vi "FIR calculator.vi"() -> ()   [LabVIEW 2015]
uses:
  <vilib>/measure/NI_MAPro.lvlib
panel:
  out "sum":dbl format="%#_18g"
  in  "COEFFICIENTVECTOR 3":string="-1, 4, 16, 32, -64, 136, -352, 1312,-352, 136, -64, 32, -16, 4, -1"
  out "CIC normalized gain":dbl[](graph)
  in  "Number of stages":i32=3
  in  "CIC input bits":i32
  out "CIC output bits":dbl[](graph)
  out "Waveform Graph 3":cluster{dbl, "df":dbl, "Mag H(w)":dbl[]}(graph)
  in  "COEFFICIENTVECTOR 2":string="-1, 4, 16, 32, -64, 136, -352, 1312,-352, 136, -64, 32, -16, 4, -1"
  out "df":dbl format="%#_6p"
  out "Waveform Graph 2":cluster{dbl, "df":dbl, "Phase H(w)":dbl[]}(graph)
  out "Waveform Graph":cluster{dbl, "df":dbl, "Mag H(w)":dbl[]}(graph)
  out "h":dbl[](array[numeric])
  in  "COEFFICIENTVECTOR1":string="-1.63744122654648e-08, -4.62216716148361e-08, -3.14335779482632e-10, 3.02310153778336e-08, 1.74890850381969e-08, 3.19482286529326e-08, -5.0994421994774e-09, -1.48653353613353e-07, -8.26761935440861e-08, 3.07015823012366e-07, 3.0080886332324e-07, -4.62653063559883e-07, -7.00184893242507e-07, 5.33506302697611e-07, 1.30813357034074e-06, -4.023225322563e-07, -2.10652650584874e-06, -7.01725431628003e-08, 3.01150223729751e-06, 1.01967031117686e-06, -3.86150372394275e-06, -2.54225818072438e-06, 4.41993348941294e-06, 4.65304341627651e-06, -4.39753212538659e-06, -7.24787717681163e-06, 3.49626558808964e-06, 1.0078701336886e-05, -1.47194685779028e-06, -1.27534942409821e-05, -1.79286233594637e-06, 1.47694078057067e-05, 6.21926306560833e-06, -1.5582846847983e-05, -1.14833577256531e-05, 1.47120230922135e-05, 1.70048621091381e-05, -1.18634714639314e-05, -2.19954283147527e-05, 7.05059419354727e-06, 2.55614060867368e-05, -6.89990820946048e-07, -2.68697800541403e-05, -6.36451714718008e-06, 2.53527750074515e-05, 1.28728450795703e-05, -2.0920846677794e-05, -1.73612517441299e-05, 1.41401071263444e-05, 1.83749862506759e-05, -6.32585991158657e-06, -1.48087387385988e-05, -4.93474951076127e-07, 6.26916256752369e-06, 3.77320372706693e-06, 6.59496436596694e-06, -8.18014683171042e-07, -2.18717457405279e-05, -1.07087232130912e-05, 3.63461490752955e-05, 3.21800806140094e-05, -4.57260582225158e-05, -6.34419626433276e-05, 4.5097399118797e-05, 0.000102325890655008, -2.96761791743105e-05, -0.00014443842428366, -4.27564702687111e-06, 0.000183291485733018, 5.84704971571537e-05, -0.000210851185795382, -0.000131721288143241, 0.000218509180683351, 0.000219358868548782, -0.000198406916678391, -0.000313120548592492, 0.000144959004714433, 0.000401644120432757, -5.63518653243416e-05, -0.000471626935842207, -6.42569578034905e-05, 0.000509602506151267, 0.000208120065222889, -0.000504183059896151, -0.000361158959377472, 0.000448371031054935, 0.000505061696434652, -0.000341847567026698, -0.0006195990988342, 0.000192428194445537, 0.000685661560487131, -1.65505528881502e-05, -0.000688880371015645, -0.000161641019845141, 0.00062329894459272, 0.000312770999488855, -0.000494493181298271, -0.000406224936898567, 0.000321490786537126, 0.000415356137374431, -0.000136895740494839, -0.000323352565488648, -1.52271175908499e-05, 0.000128983871136271, 8.38978661849253e-05, 0.000148695344532513, -1.8069608877988e-05, -0.000467701726518259, -0.000224921620006527, 0.000762940586986797, 0.000669359852735534, -0.000950271910714701, -0.00131221385225305, 0.000933507406901155, 0.00211513707866678, -0.000615289331550511, -0.00299952994722302, -8.92798158239705e-05, 0.00384566229126372, 0.00123735556393418, -0.00449671320994515, -0.00284293452198785, 0.00476808031019541, 0.00486300922613273, -0.0044617146685581, -0.00718698064468655, 0.00338458990770112, 0.00963071343738828, -0.0013698211464178, -0.0119360152269839, -0.00170150377088473, 0.0137751539824885, 0.00587879694622239, -0.0147616583115625, -0.0111272087562733, 0.014457882763948, 0.0173128033439249, -0.012382722980173, -0.0241959325972279, 0.00800309669893809, 0.031425705539797, -0.000692615375256258, -0.0385276197048089, -0.010384517623774, 0.0448576874366831, 0.0265700861070664, -0.0494359449279653, -0.050506107204478, 0.0503104495147679, 0.0885922374355363, -0.0415657042866342, -0.160704610785777, -0.00838308000357802, 0.354565700905743, 0.550459213055103, 0.354565700905743, -0.00838308000357801, -0.160704610785777, -0.0415657042866342, 0.0885922374355363, 0.0503104495147679, -0.0505061072044779, -0.0494359449279653, 0.0265700861070664, 0.0448576874366831, -0.0103845176237741, -0.0385276197048088, -0.000692615375256252, 0.031425705539797, 0.00800309669893806, -0.0241959325972279, -0.0123827229801729, 0.0173128033439249, 0.014457882763948, -0.0111272087562733, -0.0147616583115624, 0.00587879694622238, 0.0137751539824885, -0.00170150377088473, -0.0119360152269839, -0.00136982114641781, 0.00963071343738828, 0.00338458990770112, -0.00718698064468655, -0.00446171466855811, 0.00486300922613271, 0.00476808031019541, -0.00284293452198785, -0.00449671320994515, 0.00123735556393418, 0.00384566229126372, -8.92798158239772e-05, -0.00299952994722302, -0.000615289331550518, 0.00211513707866678, 0.000933507406901159, -0.00131221385225306, -0.000950271910714696, 0.000669359852735537, 0.000762940586986796, -0.00022492162000653, -0.000467701726518248, -1.80696088779863e-05, 0.0001486953445325, 8.38978661849229e-05, 0.000128983871136272, -1.5227117590845e-05, -0.000323352565488649, -0.000136895740494844, 0.000415356137374436, 0.00032149078653713, -0.000406224936898562, -0.000494493181298275, 0.000312770999488843, 0.000623298944592722, -0.000161641019845136, -0.000688880371015644, -1.6550552888178e-05, 0.000685661560487131, 0.000192428194445553, -0.0006195990988342, -0.000341847567026709, 0.000505061696434649, 0.000448371031054938, -0.000361158959377469, -0.000504183059896154, 0.000208120065222887, 0.000509602506151268, -6.42569578034892e-05, -0.000471626935842202, -5.63518653243425e-05, 0.000401644120432759, 0.000144959004714433, -0.00031312054859249, -0.000198406916678392, 0.000219358868548782, 0.00021850918068335, -0.000131721288143243, -0.000210851185795382, 5.84704971571526e-05, 0.000183291485733017, -4.27564702687076e-06, -0.000144438424283659, -2.96761791743111e-05, 0.000102325890655008, 4.50973991187948e-05, -6.34419626433272e-05, -4.57260582225145e-05, 3.21800806140092e-05, 3.63461490752936e-05, -1.07087232130911e-05, -2.18717457405289e-05, -8.18014683171156e-07, 6.59496436596684e-06, 3.77320372706711e-06, 6.26916256752231e-06, -4.93474951076179e-07, -1.48087387385992e-05, -6.32585991158642e-06, 1.83749862506765e-05, 1.41401071263443e-05, -1.73612517441294e-05, -2.09208466777939e-05, 1.28728450795703e-05, 2.53527750074514e-05, -6.36451714717938e-06, -2.68697800541402e-05, -6.8999082094604e-07, 2.55614060867367e-05, 7.05059419354764e-06, -2.19954283147527e-05, -1.18634714639311e-05, 1.70048621091382e-05, 1.47120230922136e-05, -1.14833577256531e-05, -1.55828468479833e-05, 6.21926306560826e-06, 1.47694078057067e-05, -1.79286233594635e-06, -1.27534942409822e-05, -1.47194685779027e-06, 1.00787013368863e-05, 3.49626558808964e-06, -7.2478771768118e-06, -4.39753212538663e-06, 4.65304341627645e-06, 4.41993348941295e-06, -2.54225818072432e-06, -3.86150372394272e-06, 1.01967031117682e-06, 3.01150223729752e-06, -7.01725431628033e-08, -2.10652650584875e-06, -4.02322532256309e-07, 1.30813357034074e-06, 5.33506302697589e-07, -7.00184893242498e-07, -4.62653063559866e-07, 3.0080886332324e-07, 3.07015823012349e-07, -8.26761935440843e-08, -1.48653353613346e-07, -5.09944219947347e-09, 3.19482286529264e-08, 1.74890850381962e-08, 3.02310153778422e-08, -3.14335779482123e-10, -4.62216716148339e-08, -1.63744122654657e-08"
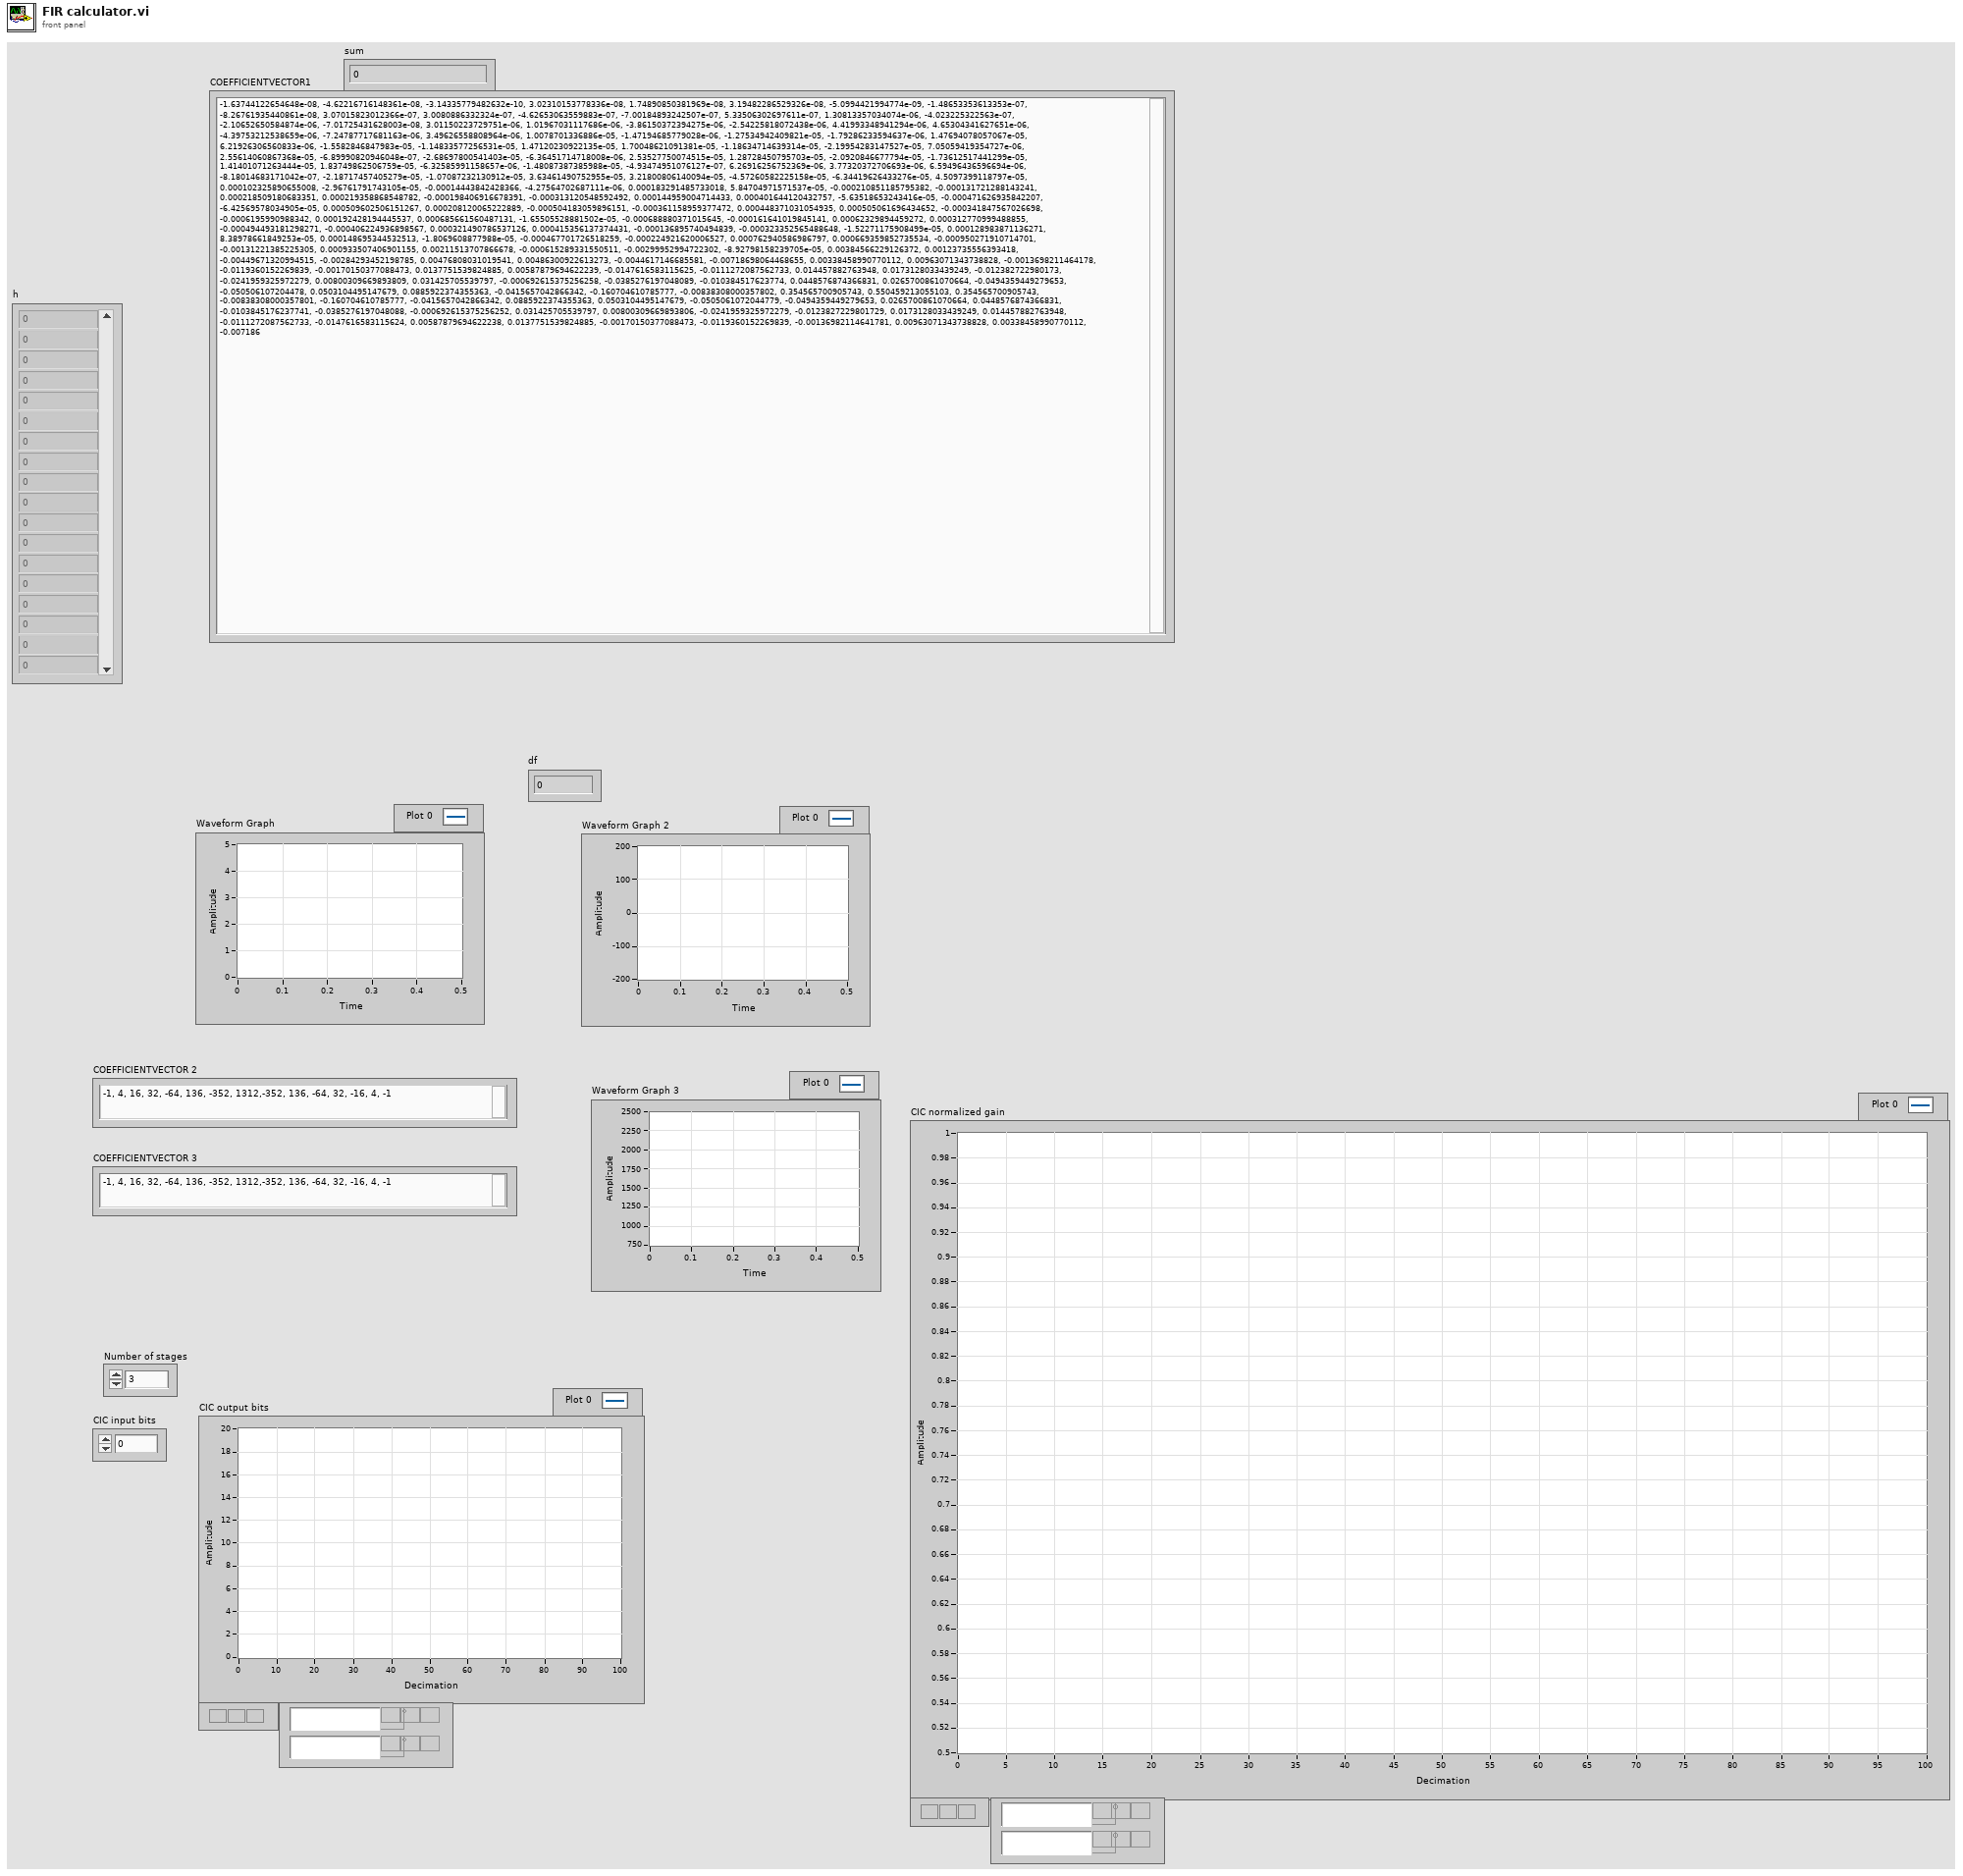
[diagram p1: front panel]
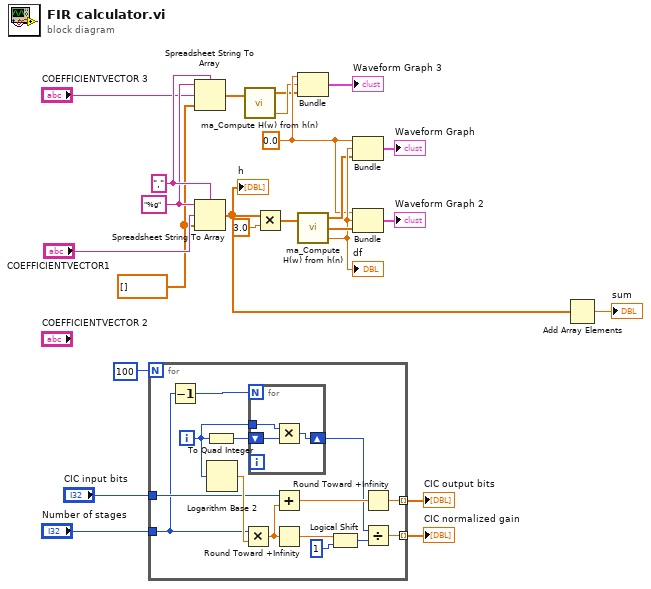
[diagram p0: block diagram]
diagram:
  w16 = 0.0
  w18 = "%g" ("format string")
  w19 = "," ("delimiter (Tab)")
  w17 = dbl[] [] ("h")
  n1 = for {
    N: 100 -> [_]
    tunnel: "Number of stages" -> [w35]
    tunnel: "CIC input bits" -> [w37]
    tunnel: [w32] -> w5 mode=indexing
    tunnel: [w29] -> w4 mode=indexing
    i -> [w34]
    n2 = Decrement(x=w35) -> (x-1=w33:i32)
    n3 = To Quad Integer(1:w34) -> (0:w25:i64)
    n4 = Logarithm Base 2(1:w34) -> (0:w38:dbl)
    n5 = Multiply(x=w35, y=w38) -> (x*y=w28:dbl)
    n6 = for {
      N: w33 -> [_]
      shift-right: [w39] -> w26
      shift-left: w25 -> [w41]
      tunnel: w34 -> [w40]
      n7 = Multiply(x=w40, y=w41) -> (x*y=w39:i64)
    }
    n8 = Add(x=w37, y=w28) -> (x+y=w36:dbl)
    n9 = Round Toward +Infinity(x=w28) -> (ceil(x): smallest int >= x=w27:dbl)
    n10 = Logical Shift(y=w27, x=1) -> (x << y=w30:i32)
    n11 = Round Toward +Infinity(x=w36) -> (ceil(x): smallest int >= x=w32:dbl)
    n12 = Divide(x=w26, y=w30) -> (x/y=w29:dbl)
  }
  "CIC output bits" <- w5
  "CIC normalized gain" <- w4
  n13 = Spreadsheet String To Array(delimiter (Tab)=w19, format string=w18, spreadsheet string="COEFFICIENTVECTOR 3", array type (2D Dbl)=w17) -> (array=w13:dbl[])
  n14 = Spreadsheet String To Array(delimiter (Tab)=w19, format string=w18, spreadsheet string="COEFFICIENTVECTOR1", array type (2D Dbl)=w17) -> (array=w2:dbl[])
  "h" <- w2
  n15 = call <vilib>:"ma_Compute H(w) from h(n).vi"("h"=w13) -> ("Mag H(w)"=w14:dbl[], "df"=w15:dbl)  [unwired: 1 in, 1 out]
  n16 = Multiply(x=w2, y=3.0) -> (x*y=w11:dbl[])
  n17 = Bundle(w16, "df"=w15, "Mag H(w)"=w14) -> (→"Waveform Graph 3":cluster{dbl, "df":dbl, "Mag H(w)":dbl[]})  [unwired: 1 in]
  n18 = call <vilib>:"ma_Compute H(w) from h(n).vi"("h"=w11) -> ("Mag H(w)"=w21:dbl[], "Phase H(w)"=w23:dbl[], "df"=w22:dbl)  [unwired: 1 in]
  "df" <- w22
  n19 = Bundle(w16, "df"=w22, "Mag H(w)"=w21) -> (→"Waveform Graph":cluster{dbl, "df":dbl, "Mag H(w)":dbl[]})  [unwired: 1 in]
  n20 = Bundle(w16, "df"=w22, "Phase H(w)"=w23) -> (→"Waveform Graph 2":cluster{dbl, "df":dbl, "Phase H(w)":dbl[]})  [unwired: 1 in]
  n21 = Add Array Elements(numeric array=w2) -> (sum=→"sum":dbl)
